vi "sub vi - GET ALL TEMP v7.vi"(0 "LA01-EN":bool, 1 "simulate":bool, 5 "LA02-EN":bool, 7 "LA03-EN":bool, 9 "LA04-EN":bool, 11 "LA05-EN":bool, 12 "Gen Cal Value":dbl) -> (2 "LOOP TIME":dbl, 3 "ID":T1, 4 "LA01 TEMP":T2, 6 "LA02 TEMP":T2, 8 "LA03 TEMP":T2, 10 "LA04 TEMP":T2, 14 "error":bool, 15 "LA05 TEMP":T2)   [LabVIEW 2013]
uses:
  program files/Global display 4.vi
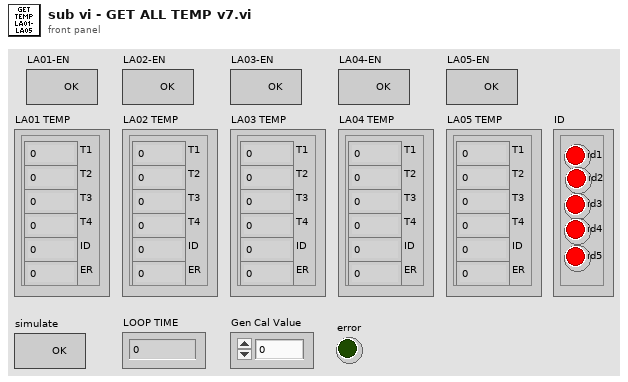
[diagram p1: front panel]
types:
  T1 = cluster{"id1":bool, "id2":bool, "id3":bool, "id4":bool, "id5":bool}
  T2 = cluster{"T1":dbl, "T2":dbl, "T3":dbl, "T4":dbl, "ID":dbl, "ER":dbl}
  T3 = cluster{"1 TL":dbl, "1 TN":dbl, "2 TL":dbl, "2 TN":dbl, "ID":dbl, "ER":dbl}
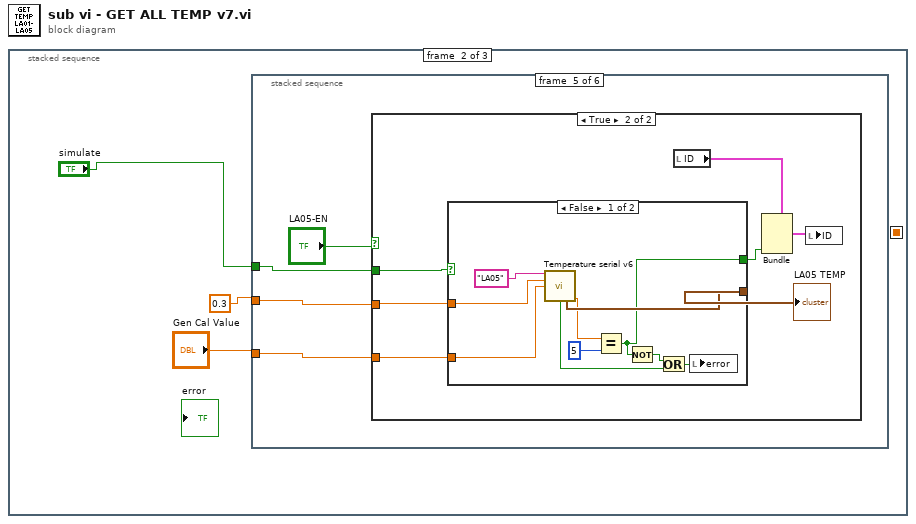
[diagram p0: block diagram]
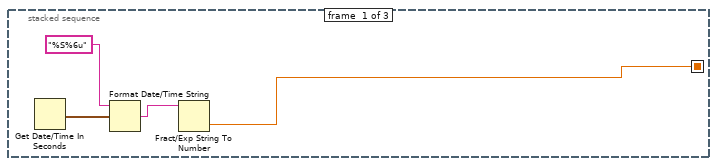
[diagram p2: hidden frame]
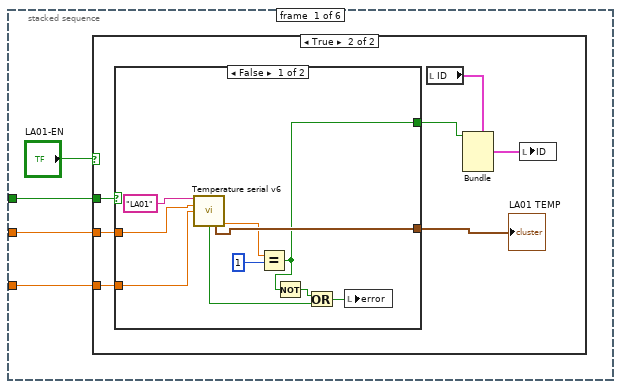
[diagram p3: hidden frame]
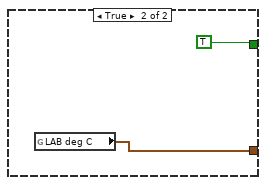
[diagram p5: hidden frame]
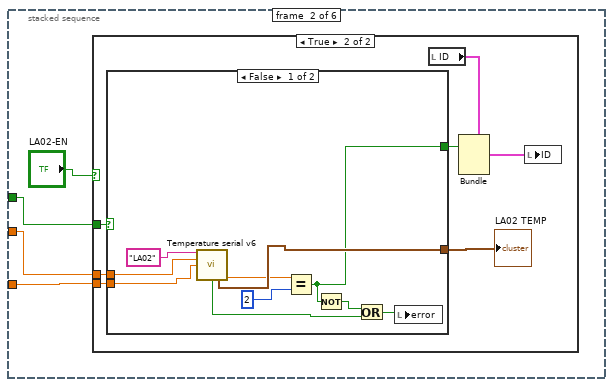
[diagram p6: hidden frame]
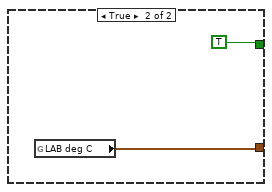
[diagram p8: hidden frame]
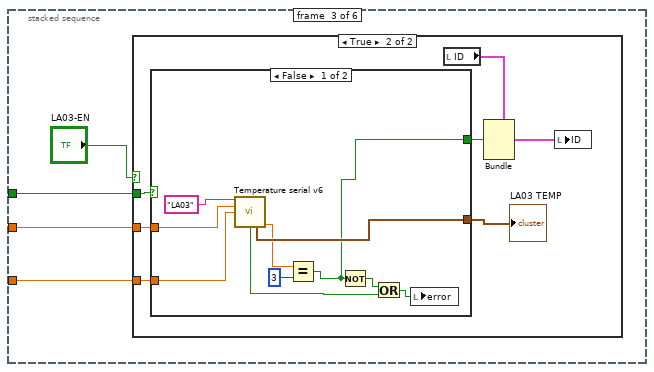
[diagram p9: hidden frame]
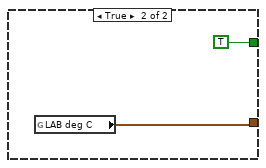
[diagram p11: hidden frame]
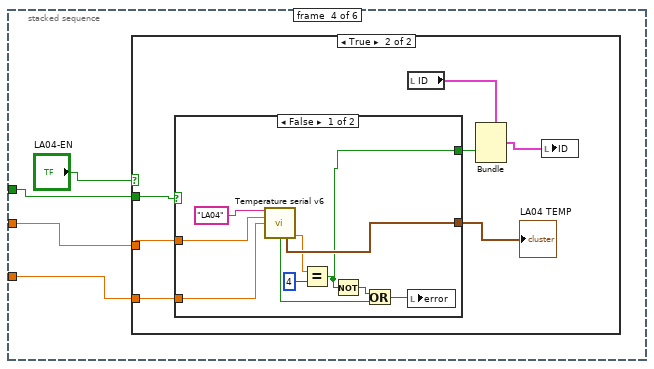
[diagram p12: hidden frame]
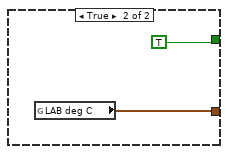
[diagram p14: hidden frame]
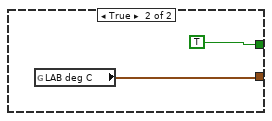
[diagram p16: hidden frame]
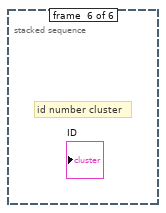
[diagram p17: hidden frame]
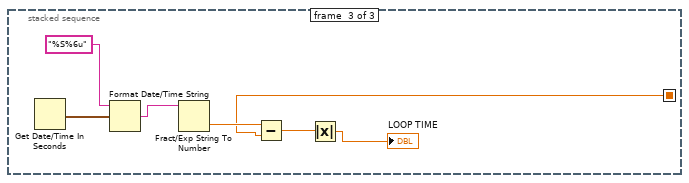
[diagram p18: hidden frame]
diagram:
  n1 = stacked-sequence {
    seq-local: [w1 _ _] -> [_ _ w125]
    frame #0 {
      n2 = Get Date/Time In Seconds() -> (seconds since 1Jan1904=w4:timestamp)
      n3 = Format Date/Time String(time format string (%c)="%S%6u", seconds (now)=w4) -> (date/time string=w2:string)  [unwired: 1 in]
      n4 = Fract/Exp String To Number(string=w2) -> (number=w1:dbl)  [unwired: 3 in, 1 out]
    }
    frame #1 {
      n5 = stacked-sequence {
        tunnel: 0.3 -> [w11 w34 w57 w80 w103 _]
        tunnel: "Gen Cal Value" -> [w10 w33 w56 w79 w102 _]
        tunnel: "simulate" -> [w8 w31 w54 w77 w100 _]
        frame #0 {
          n6 = case shown="True" "LA01-EN" {
            tunnel: w11 -> [_ w18]
            tunnel: w10 -> [_ w17]
            tunnel: w8 -> [_ w15]
            frame False {
            }
            frame True {
              n7 = case shown="False" w15 {
                tunnel: w18 -> [w27 _]
                tunnel: w17 -> [w26 _]
                tunnel: [w25 w30] -> w16
                tunnel: [w19 TRUE] -> w14
                frame False {
                  n8 = call "Temperature serial v6.vi"("Command String"="LA01", "Time Out (S)"=w27, "CALIB"=w26) -> ("error"=w22:bool, "output cluster"=w25:cluster{dbl, dbl, dbl, dbl, i32, "error #":dbl}, "Unit ID"=w21:dbl)  [unwired: 6 in, 4 out]
                  n9 = Equal?(x=w21, y=1) -> (x = y?=w19:bool)
                  n10 = Not(x=w19) -> (.not. x?=w20:bool)
                  n11 = Or(x=w20, y=w22) -> (x .or. y?=w23:bool)
                  n12 = local write "error"(w23) -> ()
                }
                frame True {
                  n13 = global read "Global display 4.vi" "LAB deg C"() -> (w30:T3)
                }
              }
              "LA01 TEMP" <- w16
              n14 = local read "ID"() -> (w13:T1)
              n15 = Bundle(cluster=w13, "id1"=w14) -> (w12:T1)  [unwired: 4 in]
              n16 = local write "ID"(w12) -> ()
            }
          }
        }
        frame #1 {
          n17 = case shown="True" "LA02-EN" {
            tunnel: w34 -> [_ w41]
            tunnel: w33 -> [_ w40]
            tunnel: w31 -> [_ w38]
            frame False {
            }
            frame True {
              n18 = case shown="False" w38 {
                tunnel: w41 -> [w50 _]
                tunnel: w40 -> [w49 _]
                tunnel: [w48 w53] -> w39
                tunnel: [w42 TRUE] -> w37
                frame False {
                  n19 = call "Temperature serial v6.vi"("Command String"="LA02", "Time Out (S)"=w50, "CALIB"=w49) -> ("error"=w46:bool, "output cluster"=w48:cluster{dbl, dbl, dbl, dbl, i32, "error #":dbl}, "Unit ID"=w44:dbl)  [unwired: 6 in, 4 out]
                  n20 = Equal?(x=w44, y=2) -> (x = y?=w42:bool)
                  n21 = Not(x=w42) -> (.not. x?=w43:bool)
                  n22 = Or(x=w43, y=w46) -> (x .or. y?=w47:bool)
                  n23 = local write "error"(w47) -> ()
                }
                frame True {
                  n24 = global read "Global display 4.vi" "LAB deg C"() -> (w53:T3)
                }
              }
              "LA02 TEMP" <- w39
              n25 = local read "ID"() -> (w36:T1)
              n26 = Bundle(cluster=w36, "id2"=w37) -> (w35:T1)  [unwired: 4 in]
              n27 = local write "ID"(w35) -> ()
            }
          }
        }
        frame #2 {
          n28 = case shown="True" "LA03-EN" {
            tunnel: w57 -> [_ w64]
            tunnel: w56 -> [_ w63]
            tunnel: w54 -> [_ w61]
            frame False {
            }
            frame True {
              n29 = case shown="False" w61 {
                tunnel: w64 -> [w73 _]
                tunnel: w63 -> [w72 _]
                tunnel: [w71 w76] -> w62
                tunnel: [w65 TRUE] -> w60
                frame False {
                  n30 = call "Temperature serial v6.vi"("Command String"="LA03", "Time Out (S)"=w73, "CALIB"=w72) -> ("error"=w68:bool, "output cluster"=w71:cluster{dbl, dbl, dbl, dbl, i32, "error #":dbl}, "Unit ID"=w67:dbl)  [unwired: 6 in, 4 out]
                  n31 = Equal?(x=w67, y=3) -> (x = y?=w65:bool)
                  n32 = Not(x=w65) -> (.not. x?=w66:bool)
                  n33 = Or(x=w66, y=w68) -> (x .or. y?=w70:bool)
                  n34 = local write "error"(w70) -> ()
                }
                frame True {
                  n35 = global read "Global display 4.vi" "LAB deg C"() -> (w76:T3)
                }
              }
              "LA03 TEMP" <- w62
              n36 = local read "ID"() -> (w59:T1)
              n37 = Bundle(cluster=w59, "id3"=w60) -> (w58:T1)  [unwired: 4 in]
              n38 = local write "ID"(w58) -> ()
            }
          }
        }
        frame #3 {
          n39 = case shown="True" "LA04-EN" {
            tunnel: w80 -> [_ w87]
            tunnel: w79 -> [_ w86]
            tunnel: w77 -> [_ w84]
            frame False {
            }
            frame True {
              n40 = case shown="False" w84 {
                tunnel: w87 -> [w96 _]
                tunnel: w86 -> [w95 _]
                tunnel: [w94 w99] -> w85
                tunnel: [w88 TRUE] -> w83
                frame False {
                  n41 = call "Temperature serial v6.vi"("Command String"="LA04", "Time Out (S)"=w96, "CALIB"=w95) -> ("error"=w92:bool, "output cluster"=w94:cluster{dbl, dbl, dbl, dbl, i32, "error #":dbl}, "Unit ID"=w90:dbl)  [unwired: 6 in, 4 out]
                  n42 = Equal?(x=w90, y=4) -> (x = y?=w88:bool)
                  n43 = Not(x=w88) -> (.not. x?=w89:bool)
                  n44 = Or(x=w89, y=w92) -> (x .or. y?=w93:bool)
                  n45 = local write "error"(w93) -> ()
                }
                frame True {
                  n46 = global read "Global display 4.vi" "LAB deg C"() -> (w99:T3)
                }
              }
              "LA04 TEMP" <- w85
              n47 = local read "ID"() -> (w82:T1)
              n48 = Bundle(cluster=w82, "id4"=w83) -> (w81:T1)  [unwired: 4 in]
              n49 = local write "ID"(w81) -> ()
            }
          }
        }
        frame #4 {
          n50 = case shown="True" "LA05-EN" {
            tunnel: w103 -> [_ w110]
            tunnel: w102 -> [_ w109]
            tunnel: w100 -> [_ w107]
            frame False {
            }
            frame True {
              n51 = case shown="False" w107 {
                tunnel: w110 -> [w119 _]
                tunnel: w109 -> [w118 _]
                tunnel: [w117 w122] -> w108
                tunnel: [w111 TRUE] -> w106
                frame False {
                  n52 = call "Temperature serial v6.vi"("Command String"="LA05", "Time Out (S)"=w119, "CALIB"=w118) -> ("error"=w115:bool, "output cluster"=w117:cluster{dbl, dbl, dbl, dbl, i32, "error #":dbl}, "Unit ID"=w113:dbl)  [unwired: 6 in, 4 out]
                  n53 = Equal?(x=w113, y=5) -> (x = y?=w111:bool)
                  n54 = Not(x=w111) -> (.not. x?=w112:bool)
                  n55 = Or(x=w112, y=w115) -> (x .or. y?=w116:bool)
                  n56 = local write "error"(w116) -> ()
                }
                frame True {
                  n57 = global read "Global display 4.vi" "LAB deg C"() -> (w122:T3)
                }
              }
              "LA05 TEMP" <- w108
              n58 = local read "ID"() -> (w105:T1)
              n59 = Bundle(cluster=w105, "id5"=w106) -> (w104:T1)  [unwired: 4 in]
              n60 = local write "ID"(w104) -> ()
            }
          }
        }
        frame #5 {
          # "id number cluster"
        }
      }
    }
    frame #2 {
      n61 = Get Date/Time In Seconds() -> (seconds since 1Jan1904=w129:timestamp)
      n62 = Format Date/Time String(time format string (%c)="%S%6u", seconds (now)=w129) -> (date/time string=w127:string)  [unwired: 1 in]
      n63 = Fract/Exp String To Number(string=w127) -> (number=w126:dbl)  [unwired: 3 in, 1 out]
      n64 = Subtract(x=w126, y=w125) -> (x-y=w124:dbl)
      n65 = Absolute Value(x=w124) -> (abs(x)=→"LOOP TIME":dbl)
    }
  }
